vi "Save Controls.vi"(8 "Error In":errorcluster, 10 "Data":cluster{"Name":string, "Variant Data":variant}[](array[cluster]), 11 "File Path":path) -> (0 "Error Out":errorcluster)   [LabVIEW 2019]
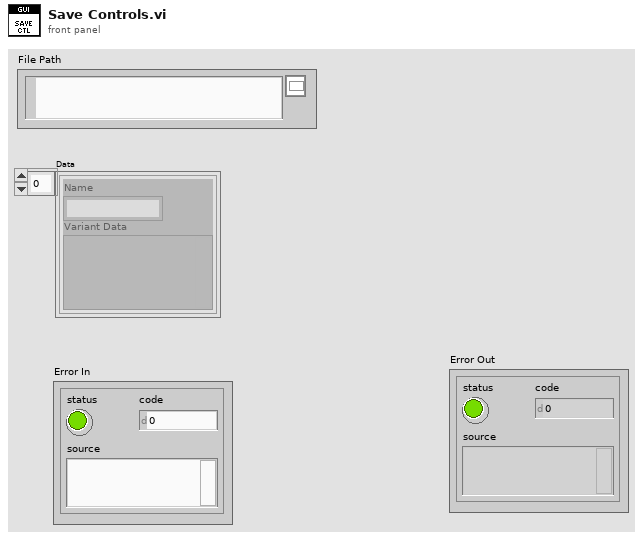
[diagram p1: front panel]
types:
  T1 = enum16{"open", "replace", "create", "open or create", "replace or create", "replace or create with confirmation"}
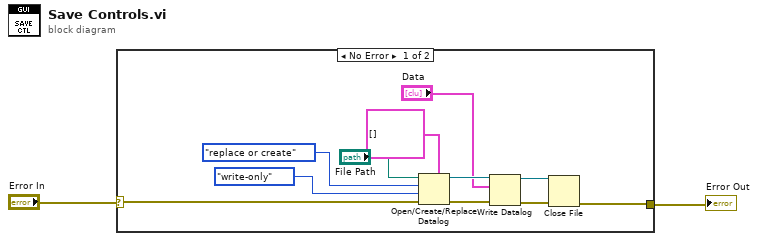
[diagram p0: block diagram]
diagram:
  n1 = case shown="No Error" "Error In" {
    selector: "Error In" -> [w4 w14]
    tunnel: [w3 w14] -> w1
    frame No Error {
      n2 = Open/Create/Replace Datalog(5:cluster{"Name":string, "Variant Data":variant}[] [] ("Control Value:Get All"), 8:w4, 9:enum16{"read/write", "read-only", "write-only"}."write-only" ("access (0:read/write)"), 10:T1."replace or create" ("operation (0:open)"), 11:"File Path") -> (0:w9:errorcluster, 3:w10:refnum<k1>)  [unwired: 1 in, 1 out]
      n3 = Write Datalog(4:w9, 6:"Data", 7:w10) -> (0:w8:errorcluster, 3:w7:refnum<k1>)
      n4 = Close File(refnum=w7, error in=w8) -> (error out=w3:errorcluster)  [unwired: 1 out]
    }
    frame Error {
    }
  }
  "Error Out" <- w1
